vi "ParseFileRows.vi"(11 "file rows":string[](array[string])) -> (3 "packages":string[][](array[string]))   [LabVIEW 2019, in "ByteLVDevEnv.lvlib"]
uses:
  ByteLVDevEnv.lvlib
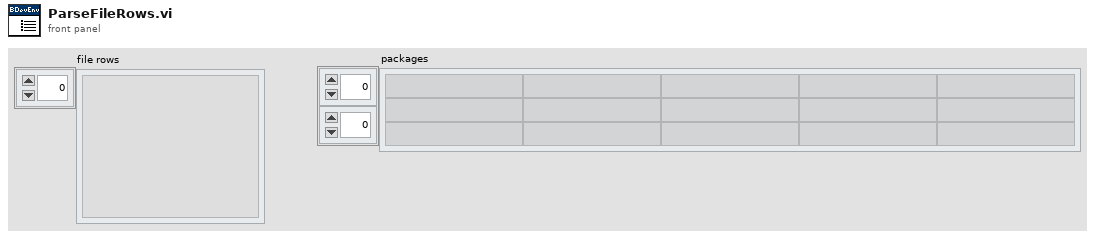
[diagram p1: front panel]
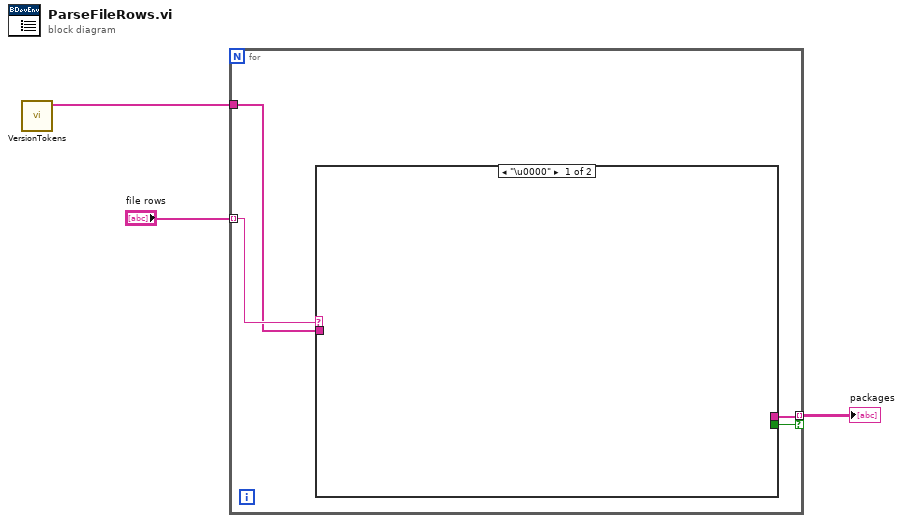
[diagram p0: block diagram]
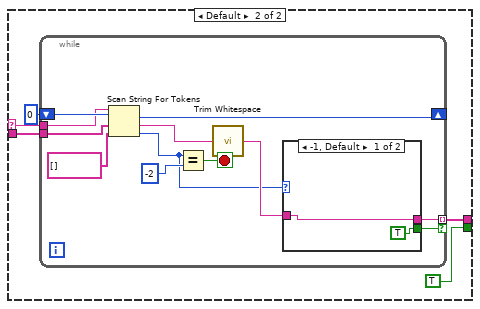
[diagram p2: hidden frame]
diagram:
  n1 = call "VersionTokens.vi"() -> ("Array"=w3:string[])  [unwired: 11 in]
  n2 = for {
    tunnel: "file rows" -> [w7] mode=indexing
    tunnel: w3 -> [w6]
    tunnel: [w5] -> w2 mode=indexing if=w4
    n3 = case shown="\"\"" w7 {
      selector: w7 -> [_ w12]
      tunnel: w6 -> [_ w11]
      tunnel: [_ w10] -> w5
      tunnel: [_ TRUE] -> w4
      frame "\u0000" {
      }
      frame Default {
        n4 = while {
          tunnel: w11 -> [w14]
          tunnel: w12 -> [w17]
          tunnel: [w19] -> w10 mode=indexing if=w16
          shift-right: [w20] -> _
          shift-left: 0 ("offset past token") -> [w21]
          stop <- w23 stop-if-true
          n5 = Scan String For Tokens(6:string[] [] ("delimiters (\\s,\\t,\\r,\\n)"), 7:w14, 8:w21, 9:w17) -> (0:w15:i32, 1:w24:string, 2:w20:i32)  [unwired: 2 in, 1 out]
          n6 = Equal?(x=w15, y=-2) -> (x = y?=w23:bool)
          n7 = call <vilib>:"Trim Whitespace.vi"("string"=w24) -> ("trimmed string"=w18:string)  [unwired: 1 in]
          n8 = case shown="-1, Default" w15 {
            tunnel: [w25 _] -> w19
            tunnel: w18 -> [w25 _]
            tunnel: [TRUE _] -> w16
            frame -1, Default {
            }
            frame -2 {
            }
          }
        }
      }
    }
  }
  "packages" <- w2
